vi "cmd_interface_test_v2.vi"() -> ()   [LabVIEW 2013]
uses:
  current_position.vi
  geometry.vi
panel:
  out "y center":dbl format="%#_13g"
  out "x limit":dbl format="%#_13g"
  out "y":dbl format="%#_13g"
  out "x":dbl format="%#_13g"
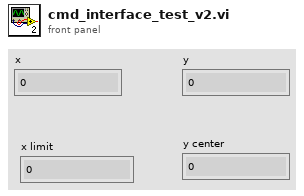
[diagram p1: front panel]
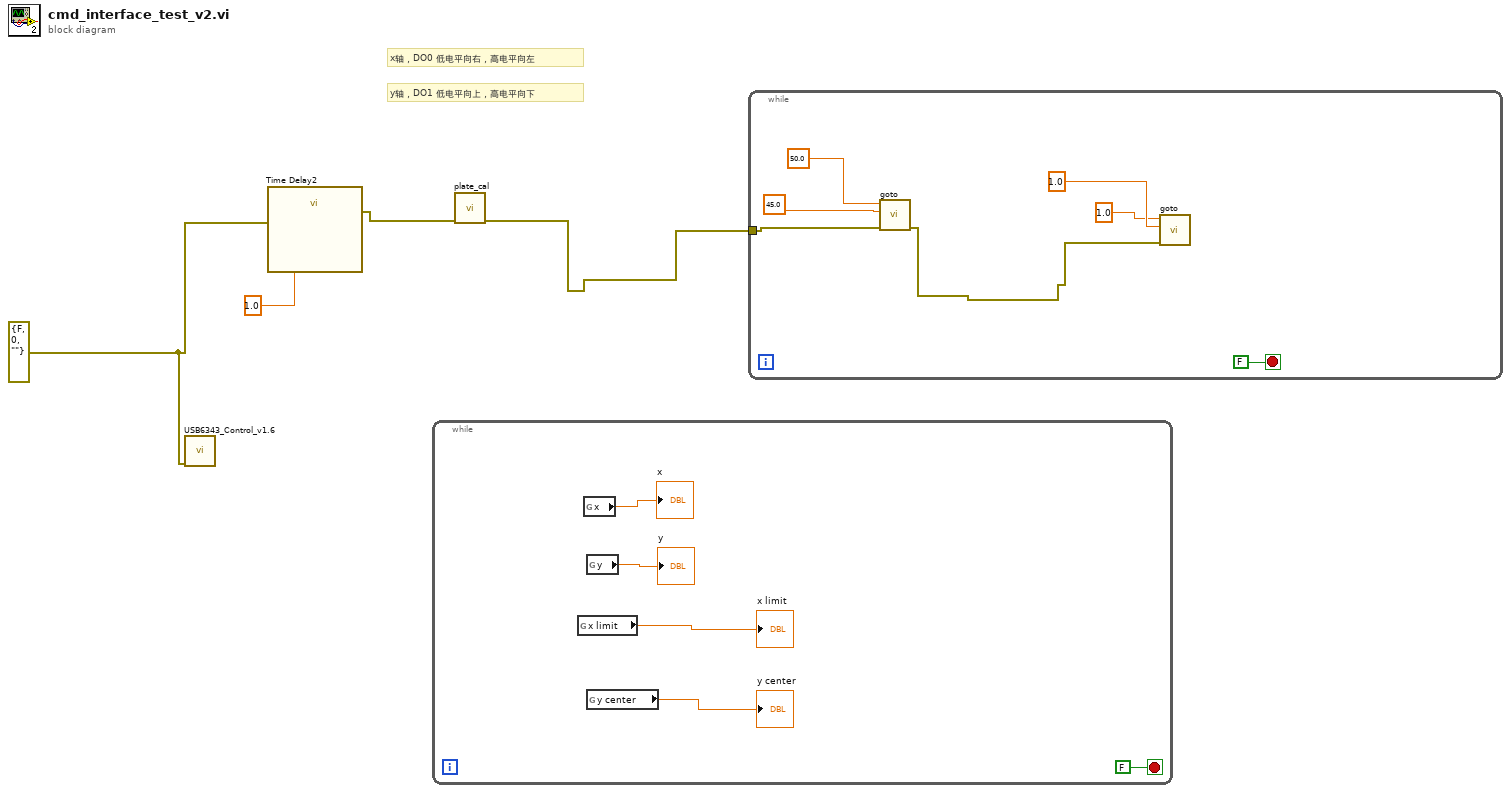
[diagram p0: block diagram]
diagram:
  w3 = errorcluster {"status"=FALSE, "code"=0, "source"=""} ("错误输出")
  # "y轴，DO1 低电平向上，高电平向下"
  # "x轴，DO0 低电平向右，高电平向左"
  n1 = call "USB6343_Control_v1.6.vi"("error in"=w3) -> ()  [unwired: 10 in, 1 out]
  n2 = call "Time Delay2"("error in (no error)"=w3, "Delay Time (s)"=1.0) -> ("error out"=w2:errorcluster)  [unwired: 9 in]
  n3 = while {
    stop <- FALSE stop-if-true
    n4 = global read "geometry.vi" "x limit"() -> (→"x limit":dbl)
    n5 = global read "current_position.vi" "x"() -> (→"x":dbl)
    n6 = global read "current_position.vi" "y"() -> (→"y":dbl)
    n7 = global read "geometry.vi" "y center"() -> (→"y center":dbl)
  }
  n8 = call "plate_cal.vi"("错误输入（无错误）"=w2) -> ("错误输出"=w1:errorcluster)  [unwired: 10 in]
  n9 = while {
    tunnel: w1 -> [w16]
    stop <- FALSE stop-if-true
    n10 = call "goto.vi"("错误输入（无错误）"=w16, "Y(mm)"=45.0, "X(mm)"=50.0) -> ("错误输出"=w10:errorcluster)  [unwired: 8 in]
    n11 = call "goto.vi"("错误输入（无错误）"=w10, "Y(mm)"=1.0, "X(mm)"=1.0) -> ()  [unwired: 8 in, 1 out]
  }
